vi "Get LR700 Formated Parameters.vi"(0 "VISA Resource Name":refnum<visa-resource-name>, 1 "Initial String":string, 4 "Channels to scan (empty - don't use scanner option)":i32[](array[numeric]), 5 "error in (no error)":errorcluster) -> (6 "Data titles":string[](array[string])=["LR700_R (Ohm)", "LR700_X (Ohm)"], 7 "Parameters":string, 8 "Time constant":dbl format="%.2f", 9 "Sensor":i32, 10 "data string":string, 11 "Local Lockout":i32, 12 "Range#":i32, 13 "Mode":i32, 14 "Range, Ohm":dbl format="%.2f", 15 "#Excitation":i32, 16 "Excitation, V":dbl format="%.2e", 17 "% of Excitation":i32, 18 "#Filter":i32, 19 "error out":errorcluster)   [LabVIEW 2015]
uses:
  GPIB/VISA  Send Receive.vi
panel:
  out "Actual Excitation, V":dbl format="%.2f"
  in  "Offset":i32
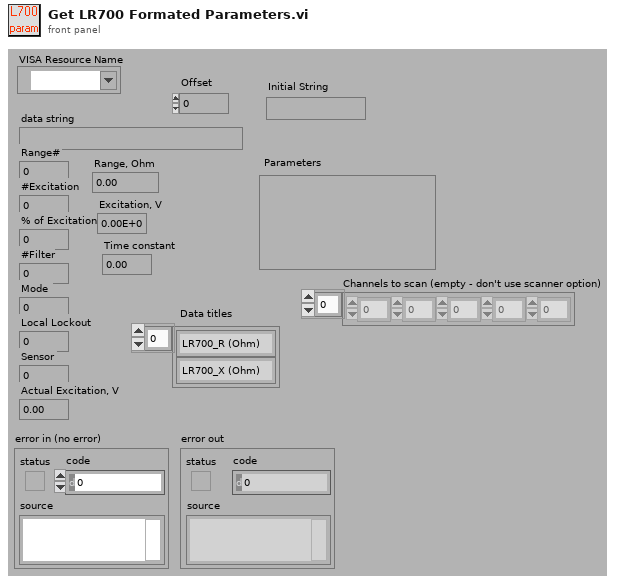
[diagram p1: front panel]
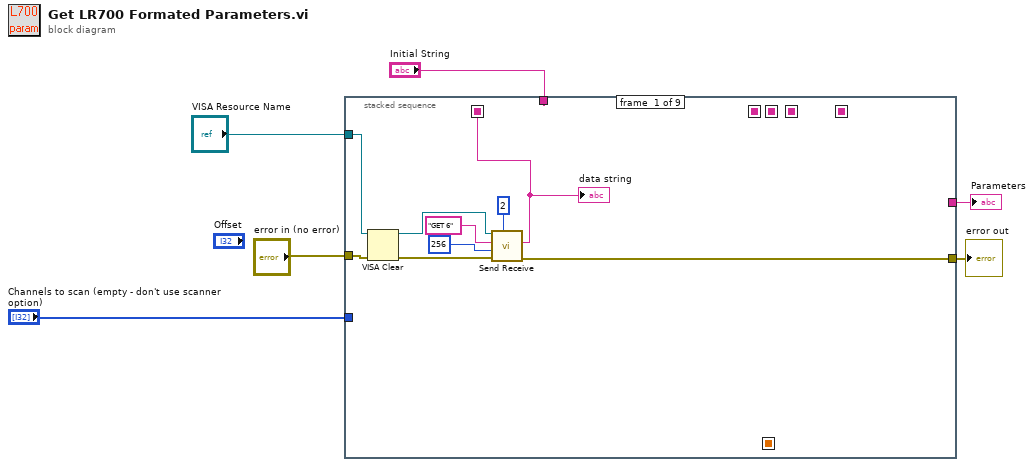
[diagram p0: block diagram]
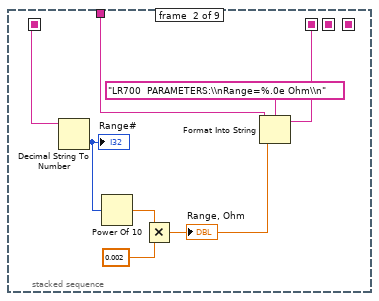
[diagram p2: hidden frame]
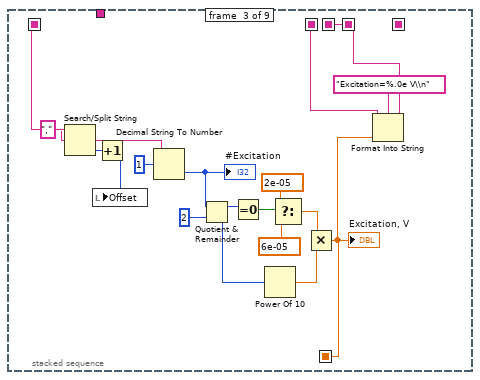
[diagram p3: hidden frame]
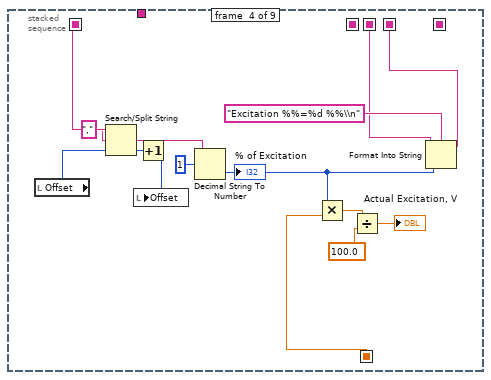
[diagram p4: hidden frame]
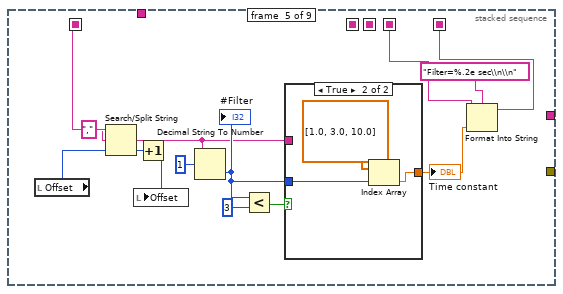
[diagram p5: hidden frame]
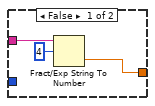
[diagram p6: hidden frame]
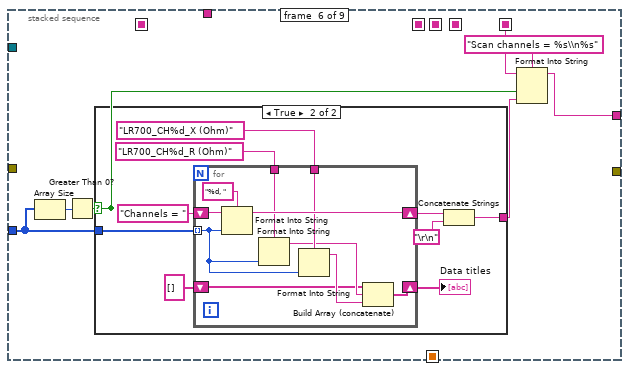
[diagram p7: hidden frame]
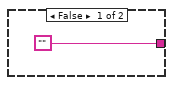
[diagram p8: hidden frame]
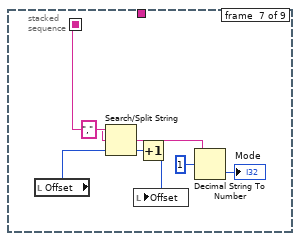
[diagram p9: hidden frame]
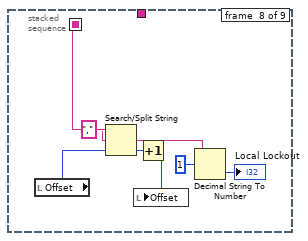
[diagram p10: hidden frame]
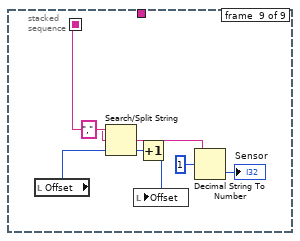
[diagram p11: hidden frame]
diagram:
  n1 = stacked-sequence {
    seq-local: [w11 _ _ _ _ _ _ _ _] -> [_ w23 w42 w57 w71 _ w112 w120 w128]
    seq-local: [_ w16 _ _ _ _ _ _ _] -> [_ _ w26 _ _ _ _ _ _]
    seq-local: [_ _ w25 _ _ _ _ _ _] -> [_ _ _ w50 _ _ _ _ _]
    seq-local: [_ _ w24 _ _ _ _ _ _] -> [_ _ _ w45 _ _ _ _ _]
    seq-local: [_ _ _ w43 _ _ _ _ _] -> [_ _ _ _ w60 _ _ _ _]
    seq-local: [_ _ _ _ w58 _ _ _ _] -> [_ _ _ _ _ w82 _ _ _]
    tunnel: [_ _ _ _ _ w78 _ _ _] -> w6
    tunnel: "Initial String" -> [_ w18 _ _ _ _ _ _ _]
    tunnel: "error in (no error)" -> [w15 _ _ _ _ _ _ _ _]
    tunnel: [w9 _ _ _ _ _ _ _ _] -> w3
    tunnel: "Channels to scan (empty - don't use scanner option)" -> [_ _ _ _ _ w84 _ _ _]
    tunnel: "VISA Resource Name" -> [w8 _ _ _ _ _ _ _ _]
    frame #0 {
      n2 = VISA Clear(VISA resource name=w8, error in (no error)=w15) -> (VISA resource name out=w7:refnum<visa-resource-name>, error out=w14:errorcluster)
      n3 = call-poly "Send Receive.vi"("Delay, ms"=u32 2, "error in (no error)"=w14, "Receive count"=256, "data string in"="GET 6", "VISA Resource Name"=w7) -> ("error out"=w9:errorcluster, "data string out"=w11:string)  [unwired: 4 in, 1 out]
      "data string" <- w11
    }
    frame #1 {
      n4 = Decimal String To Number(string=w23) -> (number=w22:i32)  [unwired: 3 out]
      "Range#" <- w22
      n5 = Power Of 10(x=w22) -> (10^x=w21:dbl)
      n6 = Multiply(x=w21, y=0.002) -> (x*y=w19:dbl)
      "Range, Ohm" <- w19
      n7 = Format Into String(format string="LR700  PARAMETERS:\\nRange=%.0e Ohm\\n", initial string=w18, w19) -> (resulting string=w16:string)  [unwired: 1 in, 1 out]
    }
    frame #2 {
      n8 = Search/Split String(string=w42, search string/char (-)="," ("search char (-)")) -> (match + rest of string=w39:string, offset of match=w38:i32)  [unwired: 2 out]
      n9 = Increment(x=w38) -> (x+1=w37:i32)
      n10 = local write "Offset"(w37) -> ()
      n11 = Decimal String To Number(string=w39, offset=1) -> (number=w36:i32)  [unwired: 2 out]
      "#Excitation" <- w36
      n12 = Quotient & Remainder(x=w36, y=2) -> (x-y*floor(x/y)=w34:i32, floor(x/y)=w30:i32)
      n13 = Equal To 0?(x=w34) -> (x = 0?=w33:bool)
      n14 = Power Of 10(x=w30) -> (10^x=w28:dbl)
      n15 = Select(t=2e-05, s=w33, f=6e-05 ("t")) -> (s? t:f=w29:dbl)
      n16 = Multiply(x=w29, y=w28) -> (x*y=w25:dbl)
      "Excitation, V" <- w25
      n17 = Format Into String(format string="Excitation=%.0e V\\n", initial string=w26, w25) -> (resulting string=w24:string)  [unwired: 1 in, 1 out]
    }
    frame #3 {
      n18 = local read "Offset"() -> (w51:i32)
      n19 = Search/Split String(string=w57, search string/char (-)="," ("search char (-)"), offset (0)=w51) -> (match + rest of string=w54:string, offset of match=w53:i32)  [unwired: 1 out]
      n20 = Increment(x=w53) -> (x+1=w52:i32)
      n21 = local write "Offset"(w52) -> ()
      n22 = Decimal String To Number(string=w54, offset=1) -> (number=w46:i32)  [unwired: 2 out]
      "% of Excitation" <- w46
      n23 = Multiply(x=w46, y=w50) -> (x*y=w49:dbl)
      n24 = Divide(x=w49, y=100.0) -> (x/y=→"Actual Excitation, V":dbl)
      n25 = Format Into String(format string="Excitation %%=%d %%\\n", initial string=w45, w46) -> (resulting string=w43:string)  [unwired: 1 in, 1 out]
    }
    frame #4 {
      n26 = local read "Offset"() -> (w66:i32)
      n27 = Search/Split String(string=w71, search string/char (-)="," ("search char (-)"), offset (0)=w66) -> (match + rest of string=w62:string, offset of match=w68:i32)  [unwired: 1 out]
      n28 = Increment(x=w68) -> (x+1=w67:i32)
      n29 = local write "Offset"(w67) -> ()
      n30 = Decimal String To Number(string=w62, offset=1) -> (number=w63:i32)  [unwired: 2 out]
      "#Filter" <- w63
      n31 = Less?(x=w63, y=3) -> (x < y?=w64:bool)
      n32 = case shown="True" w64 {
        tunnel: w63 -> [_ w76]
        tunnel: [w72 w75] -> w59
        tunnel: w62 -> [w74 _]
        frame False {
          n33 = Fract/Exp String To Number(string=w74, offset=4) -> (number=w72:dbl)  [unwired: 3 out]
        }
        frame True {
          n34 = Index Array(array=dbl[] [1.0, 3.0, 10.0], index=w76) -> (element=w75:dbl)
        }
      }
      "Time constant" <- w59
      n35 = Format Into String(format string="Filter=%.2e sec\\n\\n", initial string=w60, w59) -> (resulting string=w58:string)  [unwired: 1 in, 1 out]
    }
    frame #5 {
      n36 = Array Size(array=w84) -> (size(s)=w83:i32)
      n37 = Greater Than 0?(x=w83) -> (x > 0?=w80:bool)
      n38 = case shown="True" w80 {
        tunnel: w84 -> [_ w94]
        tunnel: ["" w90] -> w79
        frame False {
        }
        frame True {
          n39 = for {
            tunnel: w94 -> [w98] mode=indexing
            shift-right: [w102] -> w92
            shift-left: "Channels = " -> [w104]
            shift-right: [w99] -> w87
            shift-left: string[] [] -> [w95]
            tunnel: "LR700_CH%d_R (Ohm)" ("format string") -> [w101]
            tunnel: "LR700_CH%d_X (Ohm)" ("format string") -> [w100]
            n40 = Format Into String(format string="%d, ", initial string=w104, w98) -> (resulting string=w102:string)  [unwired: 1 in, 1 out]
            n41 = Format Into String(format string=w101, w98) -> (resulting string=w97:string)  [unwired: 2 in, 1 out]
            n42 = Format Into String(format string=w100, w98) -> (resulting string=w96:string)  [unwired: 2 in, 1 out]
            n43 = Build Array (concatenate)(w95, w97, w96) -> (w99:string[])
          }
          "Data titles" <- w87
          n44 = Concatenate Strings(w92, "\r\n") -> (w90:string)
        }
      }
      n45 = Format Into String(format string="Scan channels = %s\\n%s", initial string=w82, w80, w79) -> (resulting string=w78:string)  [unwired: 1 in, 1 out]
    }
    frame #6 {
      n46 = local read "Offset"() -> (w105:i32)
      n47 = Search/Split String(string=w112, search string/char (-)="," ("search char (-)"), offset (0)=w105) -> (match + rest of string=w109:string, offset of match=w108:i32)  [unwired: 1 out]
      n48 = Increment(x=w108) -> (x+1=w107:i32)
      n49 = local write "Offset"(w107) -> ()
      n50 = Decimal String To Number(string=w109, offset=1) -> (number=→"Mode":i32)  [unwired: 2 out]
    }
    frame #7 {
      n51 = local read "Offset"() -> (w113:i32)
      n52 = Search/Split String(string=w120, search string/char (-)="," ("search char (-)"), offset (0)=w113) -> (match + rest of string=w117:string, offset of match=w116:i32)  [unwired: 1 out]
      n53 = Increment(x=w116) -> (x+1=w115:i32)
      n54 = local write "Offset"(w115) -> ()
      n55 = Decimal String To Number(string=w117, offset=1) -> (number=→"Local Lockout":i32)  [unwired: 2 out]
    }
    frame #8 {
      n56 = local read "Offset"() -> (w121:i32)
      n57 = Search/Split String(string=w128, search string/char (-)="," ("search char (-)"), offset (0)=w121) -> (match + rest of string=w125:string, offset of match=w124:i32)  [unwired: 1 out]
      n58 = Increment(x=w124) -> (x+1=w123:i32)
      n59 = local write "Offset"(w123) -> ()
      n60 = Decimal String To Number(string=w125, offset=1) -> (number=→"Sensor":i32)  [unwired: 2 out]
    }
  }
  "Parameters" <- w6
  "error out" <- w3
